vi "Ch3DeconEngineFGV.vi"(8 "Error In":errorcluster, 10 "action(read)":enum16{"write", "read"}(ring)=enum."read", 11 "Ch3DeconEngine in":refnum<class "LaguerreDeconEngineClass.lvclass">) -> (0 "Error Out":errorcluster, 3 "Ch3DeconEngine out":refnum<class "LaguerreDeconEngineClass.lvclass">)   [LabVIEW 2020]
uses:
  LaguerreDeconLib/DeconEngineClass/LaguerreDeconEngineClass.lvclass
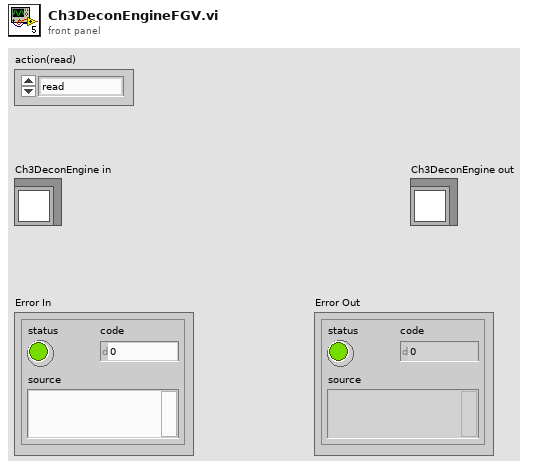
[diagram p1: front panel]
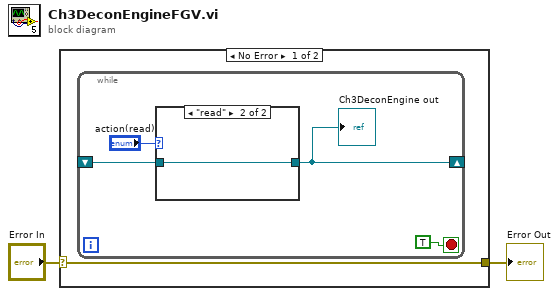
[diagram p0: block diagram]
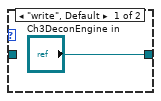
[diagram p2: hidden frame]
diagram:
  n1 = case shown="No Error" "Error In" {
    selector: "Error In" -> [w3 w10]
    tunnel: [w3 w10] -> w1
    frame No Error {
      n2 = while {
        shift-right: [w6] -> _
        shift-left: _ -> [w4]
        stop <- TRUE stop-if-true
        n3 = case shown="\"read\"" "action(read)" {
          tunnel: ["Ch3DeconEngine in" w9] -> w6
          tunnel: w4 -> [_ w9]
          frame "write", Default {
          }
          frame "read" {
          }
        }
        "Ch3DeconEngine out" <- w6
      }
    }
    frame Error {
    }
  }
  "Error Out" <- w1
